vi "SDCP SMF Receiver and Transmitter - Read Trace File.vi"(3 "error in (no error)":errorcluster, 4 "Trace File Path":path=path "E:/Projects/System Diagnostics and Control Protocol/SDCP_LabVIEW/temp/Trace Files/21 Apr 2024 20-17.csv", 5 "Parameter file path":path=path "E:/Projects/System Diagnostics and Control Protocol/SDCP_LabVIEW/Parameter Files/Motion_Processing.param") -> (0 "error out":errorcluster, 1 "Framewise output":cluster{"Data":string[][]}[](array[cluster]), 2 "Net Output":string[][](array[string]))   [LabVIEW 2020]
uses:
  Typedefs/SDCP - Standard Message Frame Parameters - FGV - commands.ctl
  <vilib>/Utility/file.llb/Read Delimited Spreadsheet (string).vi
  <vilib>/Utility/file.llb/Write Delimited Spreadsheet (string).vi
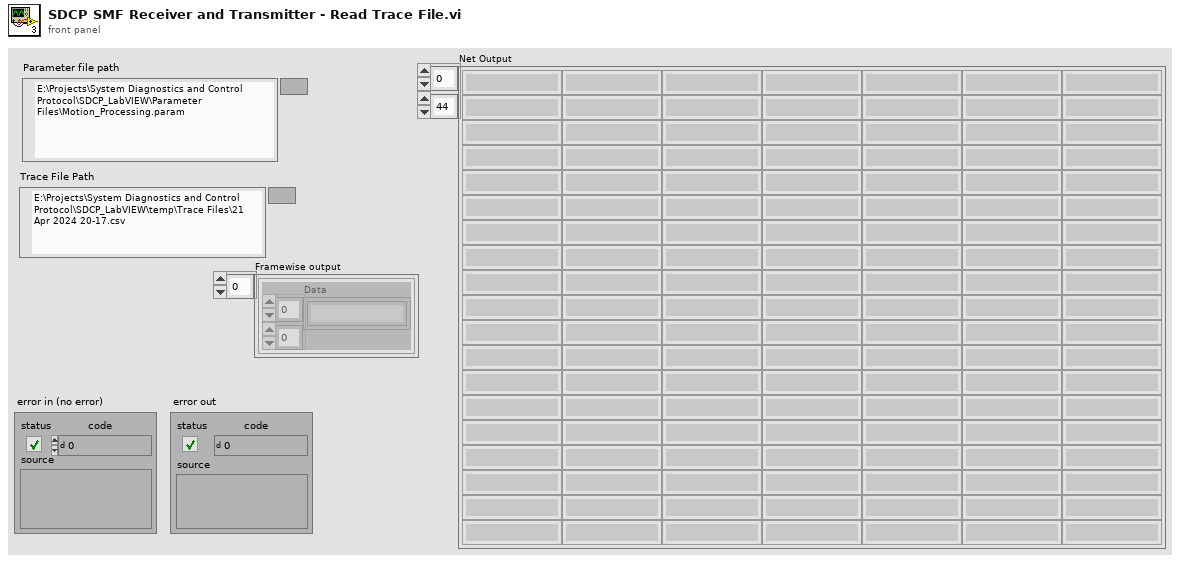
[diagram p1: front panel]
types:
  T1 = cluster{"Data bytes":u8[], "Time (ms)":dbl, "Frame ID":i32}
  T2 = cluster{"Frame ID":i32, "Data":cluster{"Data bytes":u8[], "Time (ms)":dbl}[]}
  T3 = typedef "SDCP - Standard Message Frame Parameters - FGV - commands.ctl" = enum16{"Write descriptors", "Read descriptors", "Read values", "Load parameters from file", "Write values"}
  T4 = typedef "SDCP - SMF parameter descriptors.ctl" = cluster{"Frame name":string, "Frame ID":i32, "Data type":string, "Start Position":i32, "Length":i32, "Factor":dbl, "Offset":dbl, "Parameter name":string, "Value":string}
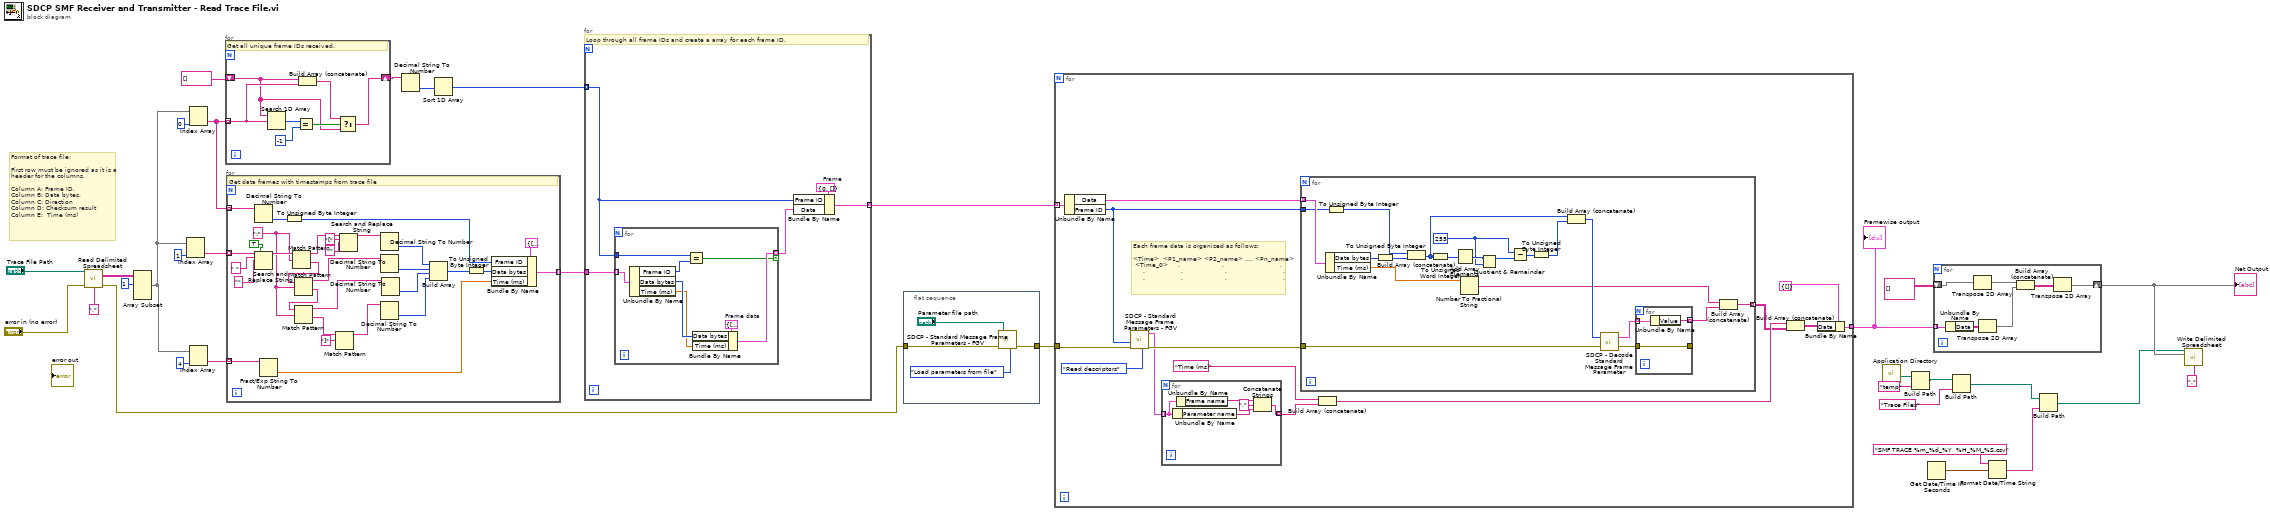
[diagram p0: block diagram]
diagram:
  # "Format of trace file:\n\nFirst row must be ignored as it is a\nheader for the columns.\n\nColumn A: Frame ID.\nColumn B: Data bytes.\nColumn C: Direction\nColumn D: Checksum result\nColumn E:  Time (ms)"
  n1 = call-poly <vilib>:"Read Delimited Spreadsheet.vi"("file path (dialog if empty)"="Trace File Path", "error in (no error)"="error in (no error)", "delimiter (\\t)"="," ("delimiter (\\t)")) -> ("all rows"=w29:string[][], "error out"=w16:errorcluster)  [unwired: 7 in, 4 out]
  n2 = Array Subset(array=w29, index (row)=1 ("index")) -> (w22:string[][])  [unwired: 3 in]
  n3 = Index Array(array=w22, index (col)=1 ("disabled index (col)")) -> (element=w23:string[])  [unwired: 1 in]
  n4 = Index Array(array=w22, index (col)=4 ("disabled index (col)")) -> (element=w20:string[])  [unwired: 1 in]
  n5 = Index Array(array=w22, index (col)=0 ("disabled index (col)")) -> (element=w19:string[])  [unwired: 1 in]
  n6 = for {
    tunnel: w19 -> [w37] mode=indexing
    shift-right: [w34] -> w26
    shift-left: string[] [] -> [w35]
    # "Get all unique frame IDs received."
    n7 = Search 1D Array(1D array=w35, element=w37) -> (index of element=w40:i32)  [unwired: 1 in]
    n8 = Equal?(x=w40, y=-1) -> (x = y?=w38:bool)
    n9 = Build Array (concatenate)(w35, w37) -> (w36:string[])
    n10 = Select(t=w36, s=w38, f=w35) -> (s? t:f=w34:string[])
  }
  n11 = for {
    tunnel: w23 -> [w50] mode=indexing
    tunnel: w20 -> [w46] mode=indexing
    tunnel: [w44] -> w17 mode=indexing
    tunnel: w19 -> [w43] mode=indexing
    w54 = ":" ("regular expression")
    # "Get data frames with timestamps from trace file"
    n12 = Decimal String To Number(string=w43) -> (number=w42:i32)  [unwired: 2 in, 1 out]
    n13 = Search and Replace String(replace all?=TRUE ("replace all? (F)"), input string=w50, search string=" ", replace string="" ("replace string (\"\")")) -> (result string=w58:string)  [unwired: 4 in, 3 out]
    n14 = Fract/Exp String To Number(string=w46) -> (number=w45:dbl)  [unwired: 3 in, 1 out]
    n15 = To Unsigned Byte Integer(number=w42) -> (unsigned 8bit integer=w41:u8)
    n16 = Match Pattern(string=w58, regular expression=w54) -> (before substring=w69:string, after substring=w59:string)  [unwired: 1 in, 2 out]
    n17 = Match Pattern(string=w59, regular expression=w54) -> (before substring=w62:string, after substring=w60:string)  [unwired: 1 in, 2 out]
    n18 = Match Pattern(string=w60, regular expression=w54) -> (before substring=w63:string, after substring=w61:string)  [unwired: 1 in, 2 out]
    n19 = Match Pattern(string=w61, regular expression="]") -> (before substring=w64:string)  [unwired: 1 in, 3 out]
    n20 = Search and Replace String(input string=w69, search string="[", replace string="" ("replace string (\"\")")) -> (result string=w70:string)  [unwired: 5 in, 3 out]
    n21 = Decimal String To Number(string=w70) -> (number=w65:i32)  [unwired: 2 in, 1 out]
    n22 = Decimal String To Number(string=w62) -> (number=w66:i32)  [unwired: 2 in, 1 out]
    n23 = Decimal String To Number(string=w64) -> (number=w68:i32)  [unwired: 2 in, 1 out]
    n24 = Decimal String To Number(string=w63) -> (number=w67:i32)  [unwired: 2 in, 1 out]
    n25 = Build Array(w65, w66, w67, w68) -> (w48:i32[])
    n26 = To Unsigned Byte Integer(number=w48) -> (unsigned 8bit integer=w47:u8[])
    n27 = Bundle By Name(cluster=T1 {"Data bytes"=[], "Time (ms)"=0.0, "Frame ID"=0}, "Frame ID"=w41, "Data bytes"=w47, "Time (ms)"=w45) -> (w44:T1)
  }
  n28 = Decimal String To Number(string=w26) -> (number=w25:i32[])  [unwired: 2 in, 1 out]
  n29 = Sort 1D Array(array=w25) -> (sorted array=w18:i32[])
  n30 = for {
    tunnel: w18 -> [w73] mode=indexing
    tunnel: w17 -> [w75]
    tunnel: [w71] -> w14 mode=indexing
    w74 = T2 {"Frame ID"=0, "Data"=[]}  # Frame
    # "Loop through all frame IDs and create a array for each frame ID."
    n31 = for {
      tunnel: w75 -> [w81] mode=indexing
      tunnel: w73 -> [w82]
      tunnel: [w77] -> w72 mode=indexing if=w76
      w80 = cluster{"Data bytes":u8[], "Time (ms)":dbl} {"Data bytes"=[], "Time (ms)"=0.0}  # Frame data
      n32 = Unbundle By Name(w81) -> ("Frame ID"=w83:i32, "Data bytes"=w79:u8[], "Time (ms)"=w78:dbl)
      n33 = Equal?(x=w82, y=w83) -> (x = y?=w76:bool)
      n34 = Bundle By Name(cluster=w80, "Data bytes"=w79, "Time (ms)"=w78) -> (w77:cluster{"Data bytes":u8[], "Time (ms)":dbl})
    }
    n35 = Bundle By Name(cluster=w74, "Frame ID"=w73, "Data"=w72) -> (w71:T2)
  }
  n36 = flat-sequence {
    tunnel: w16 -> [w87]
    tunnel: [w84] -> w15
    frame #0 {
      n37 = call "SDCP - Standard Message Frame Parameters - FGV.vi"("Parameter file path"="Parameter file path", "error in (no error)"=w87, "Command"=SDCP_-_Standard_Message_Frame_Parameters_-_FGV_-_commands."Load parameters from file") -> ("error out"=w84:errorcluster)  [unwired: 4 in, 1 out]
    }
  }
  n38 = for {
    tunnel: w15 -> [w99]
    tunnel: w14 -> [w101] mode=indexing
    tunnel: [w88] -> w13 mode=indexing
    # "Each frame data is organized as follows:\n\n<Time>  <P1_name> <P2_name> .... <Pn_name>\n <Time_0>     .                     .                            .\n     .                  .                     .                            .\n     .                  .                     .                            ."
    n39 = Unbundle By Name(w101) -> ("Data"=w100:cluster{"Data bytes":u8[], "Time (ms)":dbl}[], "Frame ID"=w96:i32)
    n40 = call "SDCP - Standard Message Frame Parameters - FGV.vi"("FID"=w96, "error in (no error)"=w99, "Command"=SDCP_-_Standard_Message_Frame_Parameters_-_FGV_-_commands."Read descriptors") -> ("SMF Parameters descriptors out"=w95:T4[], "error out"=w98:errorcluster)  [unwired: 4 in]
    n41 = for {
      tunnel: w95 -> [w106] mode=indexing
      tunnel: [w105] -> w94 mode=indexing
      n42 = Unbundle By Name(w106) -> ("Parameter name"=w102:string)
      n43 = Unbundle By Name(w106) -> ("Frame name"=w104:string)
      n44 = Concatenate Strings(w104, "." ("string"), w102) -> (w105:string)
    }
    n45 = for {
      tunnel: w100 -> [w126] mode=indexing
      tunnel: w98 -> [w125]
      tunnel: w96 -> [w123]
      tunnel: [w107] -> w91 mode=indexing
      w118 = u16 255 ("x")
      n46 = Unbundle By Name(w126) -> ("Data bytes"=w124:u8[], "Time (ms)"=w109:dbl)
      n47 = To Unsigned Byte Integer(number=w123) -> (unsigned 8bit integer=w114:u8)
      n48 = To Unsigned Byte Integer(number=w124) -> (unsigned 8bit integer=w115:u8[])
      n49 = Build Array (concatenate)(w114, w115) -> (w117:u8[])
      n50 = To Unsigned Word Integer(number=w117) -> (unsigned 16bit integer=w122:u16[])
      n51 = Add Array Elements(numeric array=w122) -> (sum=w119:u16)
      n52 = Number To Fractional String(number=w109) -> (F-format string=w108:string)  [unwired: 3 in]
      n53 = Quotient & Remainder(x=w119, y=w118) -> (x-y*floor(x/y)=w121:u16)  [unwired: 1 out]
      n54 = Subtract(x=w118, y=w121) -> (x-y=w120:u16)
      n55 = To Unsigned Byte Integer(number=w120) -> (unsigned 8bit integer=w116:u8)
      n56 = Build Array (concatenate)(w117, w116) -> (w113:u8[])
      n57 = call "SDCP - Decode Standard Message Frame Parameter.vi"("error in (no error)"=w125, "Bytes in"=w113) -> ("error out"=w111:errorcluster, "SMF Parameters out"=w112:T4[])
      n58 = for {
        tunnel: w112 -> [w129] mode=indexing
        tunnel: w111 -> [w128]
        tunnel: [w128] -> _
        tunnel: [w127] -> w110 mode=indexing
        n59 = Unbundle By Name(w129) -> ("Value"=w127:string)
      }
      n60 = Build Array (concatenate)(w108, w110) -> (w107:string[])
    }
    n61 = Build Array (concatenate)("Time (ms)", w94) -> (w92:string[])
    n62 = Build Array (concatenate)(w92, w91) -> (w89:string[][])
    n63 = Bundle By Name(cluster=cluster{"Data":string[][]} {"Data"=[]}, "Data"=w89) -> (w88:cluster{"Data":string[][]})
  }
  "Framewise output" <- w13
  n64 = call <vilib>:"Application Directory.vi"() -> ("Application Directory"=w7:path)
  n65 = Build Path(base path=w7, name or relative path="temp") -> (appended path=w5:path)
  n66 = Get Date/Time In Seconds() -> (seconds since 1Jan1904=w9:timestamp)
  n67 = for {
    tunnel: w13 -> [w135] mode=indexing
    shift-right: [w130] -> w11
    shift-left: string[][] [] -> [w136]
    n68 = Unbundle By Name(w135) -> ("Data"=w134:string[][])
    n69 = Transpose 2D Array(2D array=w136) -> (transposed array=w131:string[][])
    n70 = Transpose 2D Array(2D array=w134) -> (transposed array=w132:string[][])
    n71 = Build Array (concatenate)(w131, w132) -> (w133:string[][])
    n72 = Transpose 2D Array(2D array=w133) -> (transposed array=w130:string[][])
  }
  "Net Output" <- w11
  n73 = Build Path(base path=w5, name or relative path="Trace Files") -> (appended path=w3:path)
  n74 = Format Date/Time String(time format string (%c)="SMF TRACE %m_%d_%Y  %H_%M_%S.csv", seconds (now)=w9) -> (date/time string=w2:string)  [unwired: 1 in]
  n75 = Build Path(base path=w3, name or relative path=w2) -> (appended path=w1:path)
  n76 = call-poly <vilib>:"Write Delimited Spreadsheet.vi"("file path (dialog if empty)"=w1, "2D data"=w11, "delimiter (\\t)"="," ("delimiter (\\t)")) -> ()  [unwired: 11 in, 2 out]
